vi "Auto_calibrate.vi"(3 "Mode":T4, 5 "Traverse line":T5 {"Row Duration (mins)" format="%#.1f"; "Row No" min=0; "Trace Gas Concentration (%)" min=0.0 format="%#.2f"; "Emission Rate (l/min)" format="%#.2f"; "Tunnel Speed" format="%#.2f"; "Start X" format="%#.2f"; "Start Y" format="%#.2f"; "Start Z" format="%#.2f"; "End X" format="%#.2f"; "End Y" format="%#.2f"; "End Z" format="%#.2f"; "Averaging time (min)" min=0.0 format="%#.2f"}) -> (0 "Error Messages":string, 1 "Status":T2, 2 "Traverse Out":T5 {"Row Duration (mins)" format="%#.1f"; "Row No" min=0; "Trace Gas Concentration (%)" min=0.0 format="%#.2f"; "Emission Rate (l/min)" format="%#.2f"; "Tunnel Speed" format="%#.2f"; "Start X" format="%#.2f"; "Start Y" format="%#.2f"; "Start Z" format="%#.2f"; "End X" format="%#.2f"; "End Y" format="%#.2f"; "End Z" format="%#.2f"; "Averaging time (min)" min=0.0 format="%#.2f"})   [LabVIEW 2014]
uses:
  Gen Trav/Traverse_cluster.ctl
  Gen Trav/Spacing.ctl
  Controls/Multi_run_mode.ctl
  Controls/User_Specific_mode.ctl
  Controls/Auto_Calib_Type.ctl
  Gen Trav/Multi_Run_Status.ctl
  Controls/Auto_Calib_Case.ctl
  File/Setup_Filetype.ctl
  Calibration/Calib_mode.ctl
  Controls/Setup.ctl
  Controls/Post_Process.ctl
  Controls/Save_Data.ctl
  ADAM Client/Sub VIs/ADAM Controls/Valco_valve_ph.ctl
  Controls/App_Global.ctl
  <vilib>/Analysis/baseanly.llb/Mean (DBL).vi
  Globals/Meas_global.vi
  Globals/Calib_global.vi
  Globals/Trav_pos_global.vi
  Globals/Extra_Commands_Global.vi
  <vilib>/Analysis/NI_AALBase.lvlib
panel:
  out "Minimum St Dev":dbl[](array[numeric])
  out "Time FFID valve moved":dbl
  out "Wait factor":dbl
  out "Establishment time":string
  out "Orig Calib file string":string
  out "Concentrations":dbl[](array[numeric])
  out "FFID St Dev":dbl[][](array[numeric]) format="%.2f"
  in  "Clear Calib History":bool
  out "Coefficients":dbl[][](array[numeric]) format="%.2f"
  out "Currently in Case":T1
  out "Valve position":dbl format="%.2f"
  out "Currently On":i32
  out "Values":dbl[][](array[numeric]) format="%.2f"
  out "FF Indexes":i16[](array[numeric])
  out "Ch No's":i16[](array[numeric])
  out "No of Calib Points":i32
  out "Root Name":string[](array[string])
  out "Calibration varying":T3
  in  "stop":bool
  out "New Calib Filenames":path[](array[path])
  # "Specific Argument Options\n      Tunnel Speed;1;2;3;4\nOR  Traverse Position\nOR   Concentration"
  # "X           Y            Z"
  # "Start"
  # "End"
  # "X           Y            Z"
  # "Start"
  # "End"
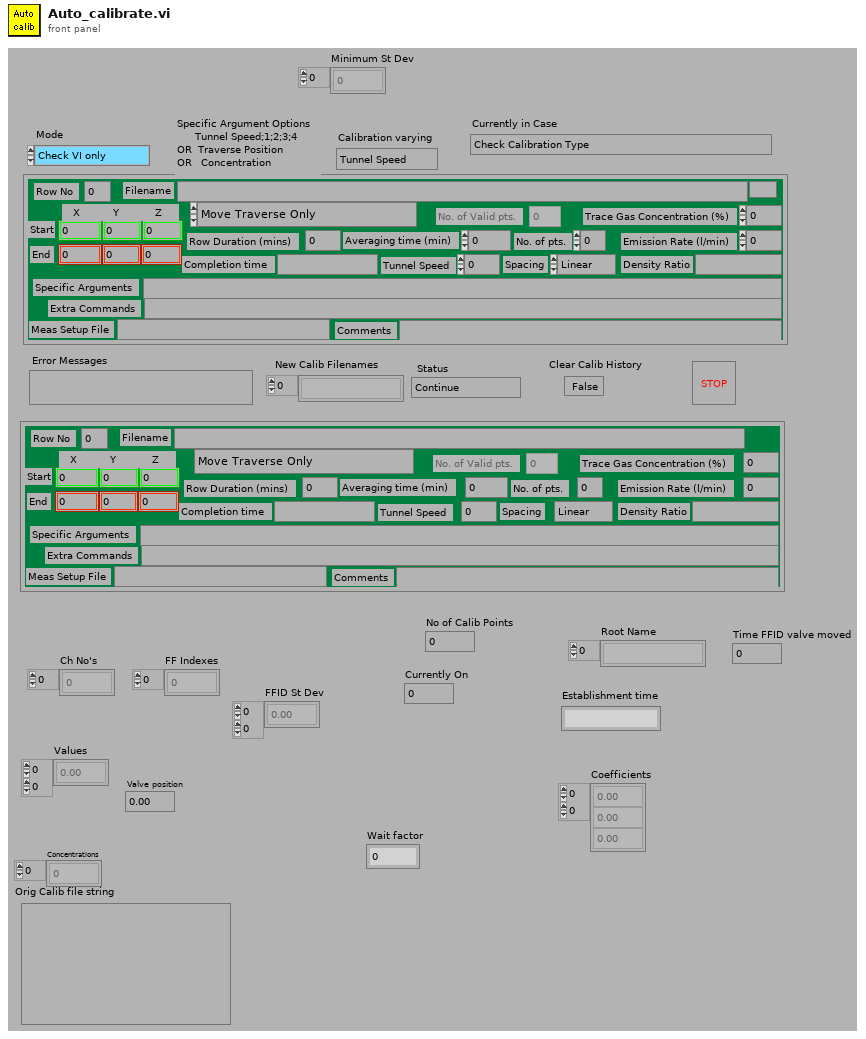
[diagram p1: front panel]
types:
  T1 = typedef "Auto_Calib_Case.ctl" = enum16{"Check Calibration Type", "Check if Original Calib file is Valid", "Get sampling rate etc. from meas setup file", "Setup Calibration Program", "Get Channel Numbers", "Check use latest selected on Mesurement setup files", "Create New Calib Filenames", "Setup Calibration Values in 2D array", "Create Measurement Setup File (Concentration Only)", "Are There Enough Calibration Points", "Set Measurement Conditions", "Measure Calibration Point", "Do Another Calibration Point?", "Skip Next Frame?", "Insert New calibration Filenames into Measurement Setup file", "Warn if FFID calibration is very non linear", "Warn if FFID variance is high", "Insert Bkgnd Variance into calib file", "Warn if FFID voltages are too low", "Warn if Current Calibration fit is poor", "Warn if Calibration Coefficients have significantly altered", "End"}
  T2 = typedef "Multi_Run_Status.ctl" = enum16{"Continue", "Jump to Next Point", "Jump to Next Row", "Jump To Fall Back", "Terminate Run"}
  T3 = typedef "Auto_Calib_Type.ctl" = enum16{"Tunnel Speed", "Traverse Position", "Concentration"}
  T4 = typedef "User_Specific_mode.ctl" = enum16{"Check VI only", "Run VI"}
  T5 = typedef "Traverse_cluster.ctl" = cluster{"Start X":dbl, "Start Y":dbl, "Start Z":dbl, "End X":dbl, "End Y":dbl, "End Z":dbl, "No. of pts.":i32, "Spacing":T6, "Filename":path, "Tunnel Speed":dbl, "Averaging time (min)":dbl, "Extra Commands":string, "Specific Arguments":string, "Emission Rate (l/min)":dbl, "Trace Gas Concentration (%)":dbl, "Density Ratio":string, "Comments":string, "Row No":i32, "Row Type Selector":T7, "Completion time":string, "Row Duration (mins)":dbl, "No. of Valid pts.":i32, "Meas Setup File":string}
  T6 = typedef "Spacing.ctl" = enum16{"Linear", "Log", "Gauss", "Specified", "N/A"}
  T7 = typedef "Multi_run_mode.ctl" = enum16{"Move Traverse Only", "Set Tunnel Speed Only", "Set Source Only", "Set Measurement Conditions", "Single Measurement", "Vertical Profile", "Lateral Profile", "Longitudinal Profile", "Explore Volume", "Multi-Axis Profile", "Auto Calibrate", "Meas Fast FID Bkgnd", "Check Beam Power", "Scanning Valve Measurement", "Run VI Named:", "Set ADAM Ch", "Wait (minutes)", "Send Message", "Synchronize With:", "Fall Back to this Row", "Turn Off Row Repeating", "Blank Row", "Traverse 3D Volume"}
  T8 = typedef "Setup_Filetype.ctl" = enum16{"Measurement Setups", "Calibration Setups", "General", "Results File Plotter Setups", "Speed Calib Tweaks"}
  T9 = typedef "Calib_mode.ctl" = enum16{"Show Setup", "Take a New Calibration Point", "Refit Curve", "Setup Front Panel"}
  T10 = typedef "Save_Data.ctl" = enum16{"Save No Data", "Save Data"}
  T11 = typedef "Post_Process.ctl" = enum16{"Take New Data", "Post Process Raw Data File"}
  T12 = typedef "Setup.ctl" = enum16{"Run Program", "Show Setup", "Save Current Setup", "Setup Front Panel"}
  T13 = typedef "App_Global.ctl" = enum16{"Read Global", "Write to Global", "Initialise Array"}
  T14 = typedef "Cal_Inst_type.ctl" = enum16{"Propeller anemometer", "Pressure Transducer", "Hot wire", "Cross wire velocity", "Cross wire angle", "Generic Linear", "Generic Polynomial", "Generic BackPoly", "Fast FID", "Thermocouple", "Cold wire", "Pulsed Wire"}
  T15 = typedef "Ref_Inst_type.ctl" = enum16{"Propellor anemometer", "Pressure Transducer", "Raw voltage", "Pitot-static tube", "Preston tube", "Generic Linear", "Generic Polynomial", "Thermocouple", "LDA", "Enter Value", "ADAM Channel"}
  T16 = cluster{"2nd Ref type":T15, "2nd inst present":bool}
  T17 = cluster{"high limit (10V)":sgl, "low limit (-10V)":sgl, "Ch No":i16, "Var name":string}[]
  T18 = cluster{"high limit (10V)":sgl, "low limit (-10V)":sgl, "Ch No":i16, "Var name":string}
  T19 = typedef "Inst_type.ctl" = enum16{"Propeller anemometer", "Raw voltage", "Pressure Transducer", "Pitot-static tube", "Preston tube", "Hot wire", "Cross wire 1", "Cross wire 2", "Generic Linear", "Generic Polynomial", "Generic BackPoly", "Fast FID", "Thermocouple", "Cold wire", "Pulsed Wire", "LDA Vel", "LDA Tran time", "LDA Arr time"}
  T20 = cluster{"high limit (10V)":sgl, "low limit (-10V)":sgl, "Ch No":i16, "Calib filename":path, "Inst type":T19, "Symbol":string, "Move channel":bool, "Use Latest":bool, "D":dbl, "Ch Name":string}[]
  T21 = typedef "Status_Cluster.ctl" = cluster{"Status":T2, "Error Type":string, "Error Description":string}
  T22 = typedef "Valco_valve_ph.ctl" = u16
  T23 = typedef "Time_Trace_Cluster.ctl" = cluster{"Weighting":dbl[], "Time (s)":dbl[], "Voltage":dbl[], "Eng Values":dbl[]}
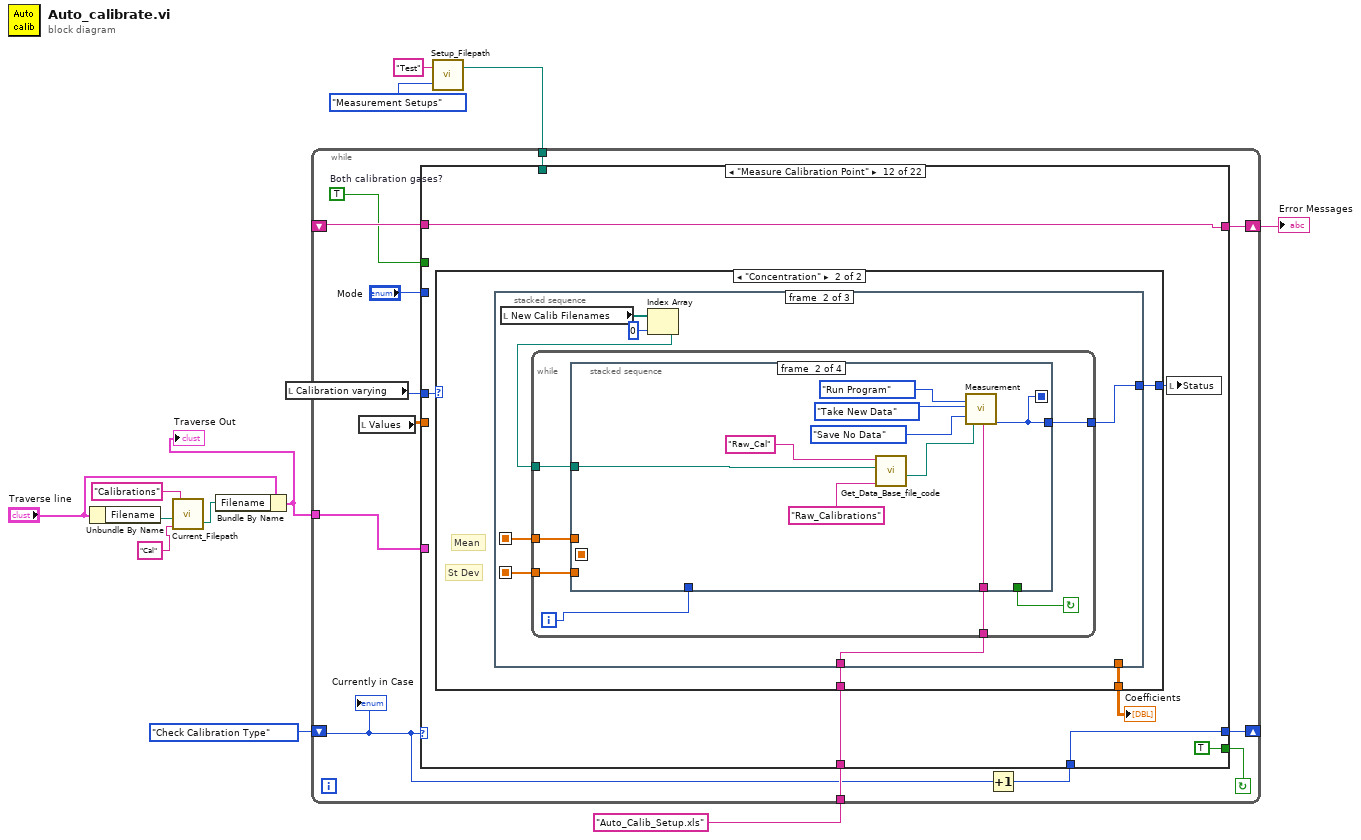
[diagram p0: block diagram]
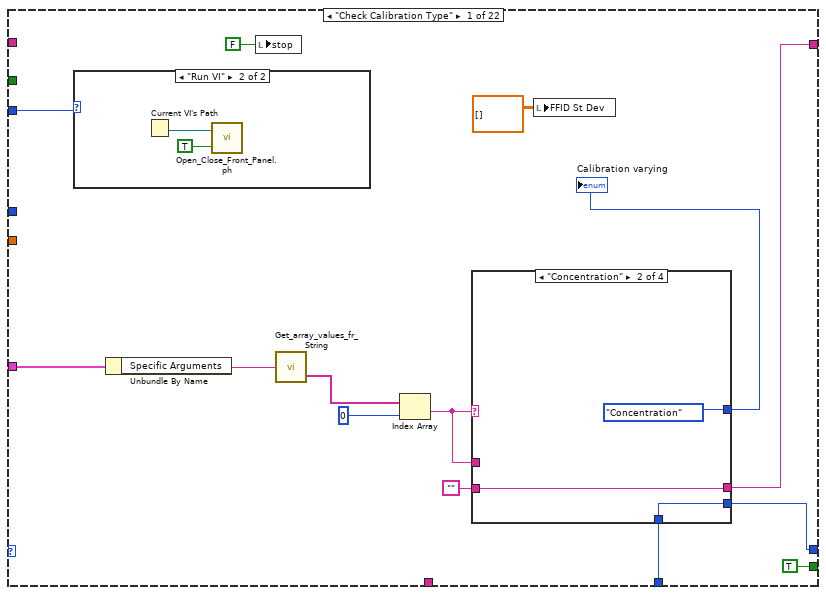
[diagram p2: hidden frame]
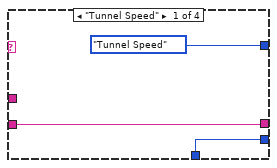
[diagram p4: hidden frame]
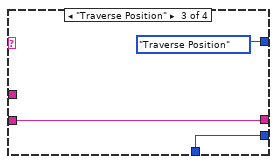
[diagram p5: hidden frame]
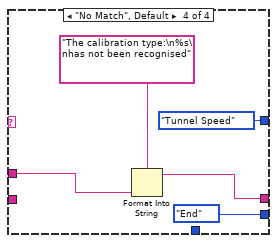
[diagram p6: hidden frame]
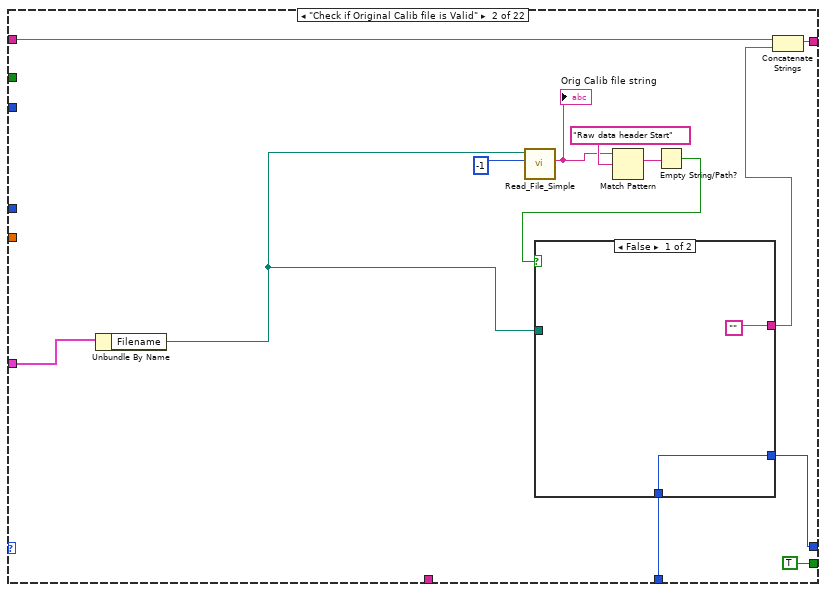
[diagram p7: hidden frame]
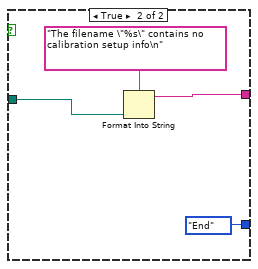
[diagram p8: hidden frame]
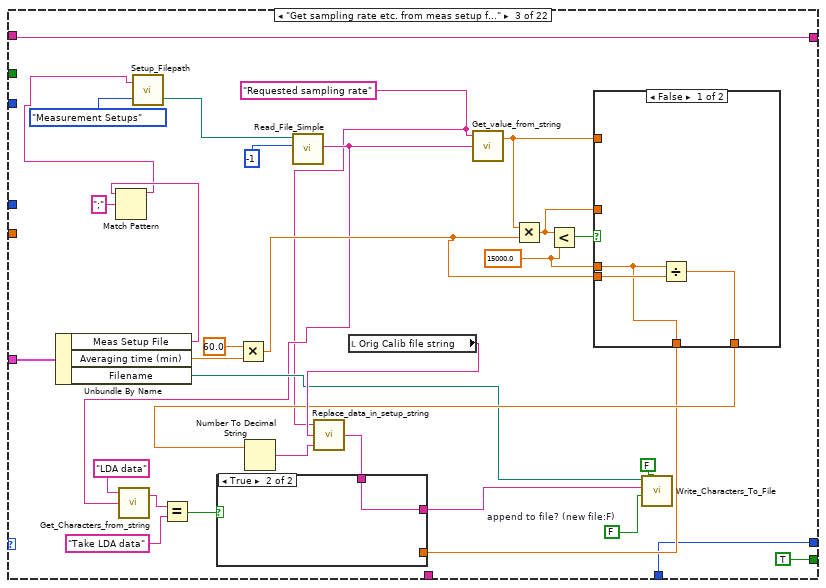
[diagram p9: hidden frame]
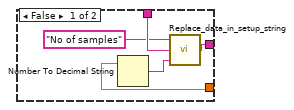
[diagram p10: hidden frame]
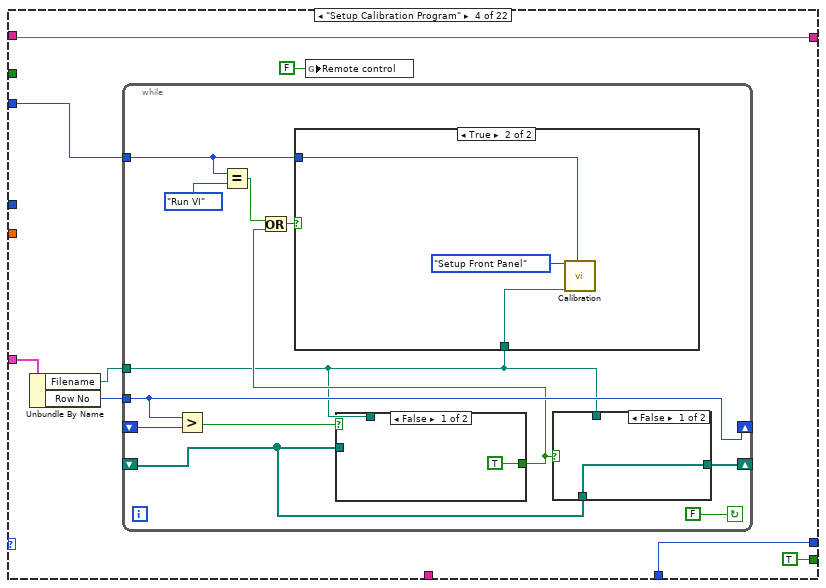
[diagram p12: hidden frame]
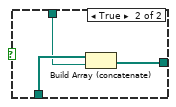
[diagram p13: hidden frame]
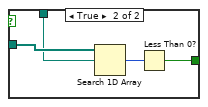
[diagram p15: hidden frame]
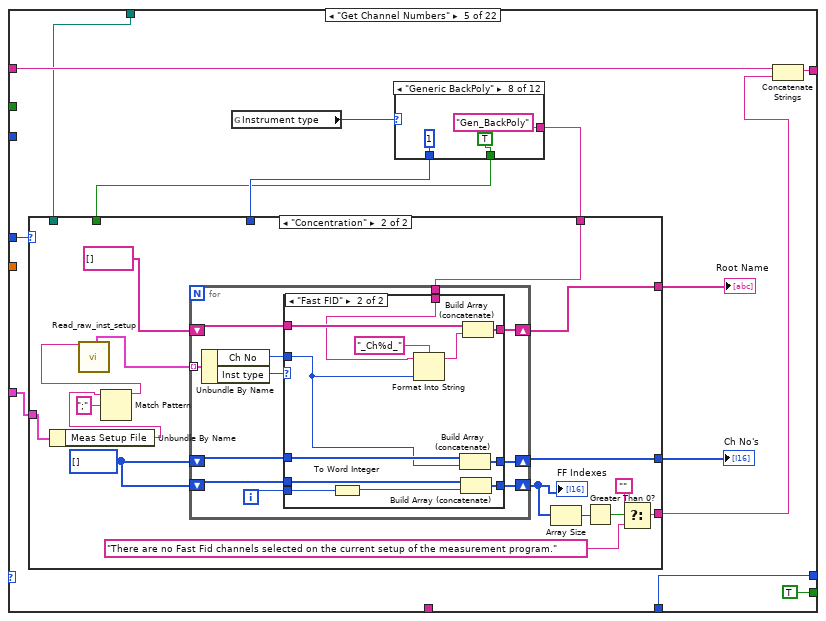
[diagram p16: hidden frame]
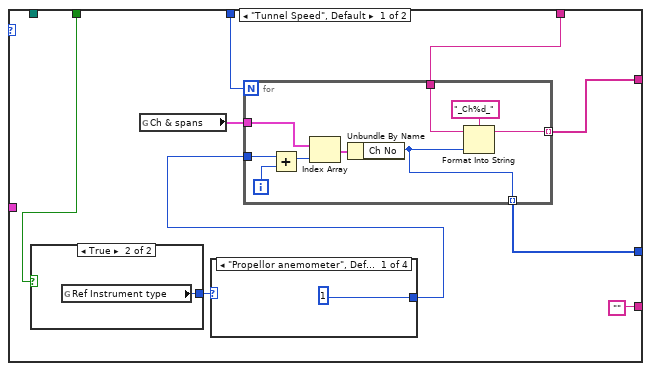
[diagram p17: hidden frame]
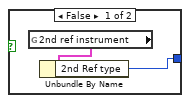
[diagram p18: hidden frame]
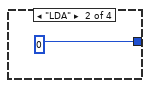
[diagram p19: hidden frame]
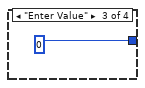
[diagram p20: hidden frame]
diagram:
  n1 = Unbundle By Name("Traverse line") -> ("Filename"=w5:path)
  n2 = call "Current_Filepath.vi"("Short_Name"="Cal" ("Data Type"), "Filename in"=w5, "Data Type"="Calibrations") -> ("Filename Out"=w4:path)  [unwired: 1 in, 1 out]
  n3 = Bundle By Name(cluster="Traverse line", "Filename"=w4) -> (w2:T5)
  "Traverse Out" <- w2
  n4 = call "Setup_Filepath.vi"("Setup File Type"=Setup_Filetype."Measurement Setups", "Filename in"="Test") -> ("Directory"=w7:path)  [unwired: 1 out]
  n5 = while {
    shift-left: _ -> [w18]
    shift-right: [w19] -> w11
    shift-left: Auto_Calib_Case."Check Calibration Type" ("Currently in Case") -> [w17]
    shift-right: [w16] -> _
    tunnel: "Auto_Calib_Setup.xls" -> [w25]
    tunnel: w7 -> [w14]
    tunnel: w2 -> [w13]
    stop <- w22 continue-if-true
    w15 = TRUE  # Both calibration gases?
    n6 = local read "Calibration varying"() -> (w21:T3)
    n7 = local read "Values"() -> (w20:dbl[][])
    n8 = Increment(x=w17) -> (x+1=w23:T1)
    n9 = case shown="\"Measure Calibration Point\"" w17 {
      tunnel: w13 -> [w39 w68 w106 w121 w152 _ w320 w375 w408 _ w575 _ _ _ _ _ _ _ _ _ w984 w1015]
      tunnel: "Mode" -> [w30 _ _ w122 _ _ w327 _ w409 _ w570 _ w728 _ _ _ _ _ _ _ _ w1016]
      tunnel: w25 -> [_ _ _ _ _ _ _ _ w413 _ _ w638 _ _ _ _ _ _ _ _ _ _]
      tunnel: [w28 w58 w88 w124 w155 w271 w324 w366 w411 w538 w563 w637 w729 w755 w767 w786 w824 w889 w907 w963 w1007 w1020] -> w16
      tunnel: w23 -> [w29 w57 w88 w124 w155 w271 w324 w367 w411 w537 w558 w637 _ w754 w766 w786 w824 w889 w907 w963 w1007 w1020]
      tunnel: [TRUE TRUE TRUE TRUE TRUE TRUE TRUE TRUE w407 TRUE TRUE TRUE TRUE TRUE TRUE TRUE TRUE TRUE TRUE TRUE TRUE FALSE] -> w22
      tunnel: w21 -> [_ _ _ _ w159 _ w323 w373 _ _ w562 w639 w727 w753 w769 _ _ _ _ _ _ w1017]
      tunnel: w20 -> [_ _ _ _ _ _ _ _ w406 w547 w574 _ _ _ _ _ w831 _ w913 _ _ _]
      tunnel: [w32 w60 w86 w125 w156 w272 w337 w370 w412 w541 w559 w635 w726 w758 w773 w795 w838 w885 w914 w952 w1000 w1019] -> w19
      tunnel: w18 -> [_ w62 w86 w125 w158 w272 w337 w369 w412 w542 w559 w635 w726 w758 w773 w795 w838 w885 w914 w952 w1000 w1019]
      tunnel: w15 -> [_ _ _ _ _ _ _ w368 _ _ _ _ _ _ _ _ _ _ _ _ _ w1014]
      tunnel: w14 -> [_ _ _ _ w151 w274 _ _ w410 _ _ _ _ _ _ _ _ _ _ _ _ _]
      frame "Check Calibration Type" {
        n10 = case shown="\"Run VI\"" w30 {
          frame "Check VI only" {
          }
          frame "Run VI" {
            n11 = Current VI's Path() -> (path=w40:path)
            n12 = call "Open_Close_Front_Panel.ph.vi"("Front Panel Window:Open"=TRUE, "VI path"=w40) -> ()  [unwired: 2 out]
          }
        }
        n13 = Unbundle By Name(w39) -> ("Specific Arguments"=w38:string)
        n14 = local write "stop"(FALSE) -> ()
        n15 = call "Get_array_values_fr_String.vi"("String Value"=w38) -> ("String array"=w37:string[])  [unwired: 1 out]
        n16 = Index Array(array=w37, index=0 ("Index")) -> (element=w35:string)
        n17 = case shown="\"Concentration\"" w35 {
          tunnel: [Auto_Calib_Type."Tunnel Speed" ("Calibration varying") Auto_Calib_Type."Concentration" ("Calibration varying") Auto_Calib_Type."Traverse Position" ("Calibration varying") Auto_Calib_Type."Tunnel Speed" ("Calibration varying")] -> w33
          tunnel: w35 -> [_ _ _ w54]
          tunnel: [w43 w46 w49 w52] -> w32
          tunnel: "" -> [w43 w46 w49 _]
          tunnel: w29 -> [w42 w45 w48 _]
          tunnel: [w42 w45 w48 Auto_Calib_Case."End" ("Currently in Case")] -> w28
          frame "Tunnel Speed" {
          }
          frame "Concentration" {
            (unwired) ""
          }
          frame "Traverse Position" {
          }
          frame "No Match", Default {
            n18 = Format Into String(format string="The calibration type:\n%s\nhas not been recognised" ("Format String"), w54) -> (resulting string=w52:string)  [unwired: 2 in, 1 out]
          }
        }
        "Calibration varying" <- w33
        n19 = local write "FFID St Dev"(dbl[][] [] ("FFID Variance")) -> ()
      }
      frame "Check if Original Calib file is Valid" {
        n20 = Unbundle By Name(w68) -> ("Filename"=w56:path)
        n21 = call "Read_File_Simple.vi"("Filename"=w56, "number of characters (all:-1)"=-1) -> ("string"=w65:string)  [unwired: 1 in, 7 out]
        "Orig Calib file string" <- w65
        n22 = Match Pattern(string=w65, regular expression="Raw data header Start") -> (match substring=w64:string)  [unwired: 4 out]
        n23 = Empty String/Path?(string/path=w64) -> (empty?=w63:bool)
        n24 = case shown="False" w63 {
          tunnel: w56 -> [_ w74]
          tunnel: ["" w72] -> w61
          tunnel: [w69 Auto_Calib_Case."End" ("Currently in Case")] -> w58
          tunnel: w57 -> [w69 _]
          frame False {
          }
          frame True {
            n25 = Format Into String(format string="The filename \"%s\" contains no calibration setup info\n" ("Format String"), w74) -> (resulting string=w72:string)  [unwired: 2 in, 1 out]
          }
        }
        n26 = Concatenate Strings(w62, w61) -> (w60:string)
      }
      frame "Get sampling rate etc. from meas setup file" {
        w89 = FALSE  # append to file? (new file:F)
        w78 = "Requested sampling rate"
        w96 = 15000.0 ("y")
        n27 = Unbundle By Name(w106) -> ("Meas Setup File"=w84:string, "Averaging time (min)"=w104:dbl, "Filename"=w91:path)
        n28 = Match Pattern(string=w84, regular expression=";") -> (before substring=w76:string)  [unwired: 4 out]
        n29 = call "Setup_Filepath.vi"("Setup File Type"=Setup_Filetype."Measurement Setups", "Filename in"=w76) -> ("Filename Out"=w75:path)  [unwired: 1 out]
        n30 = Multiply(x=60.0, y=w104) -> (x*y=w95:dbl)
        n31 = call "Read_File_Simple.vi"("Filename"=w75, "number of characters (all:-1)"=-1) -> ("string"=w83:string)  [unwired: 1 in, 7 out]
        n32 = call "Get_Characters_from_string.vi"("Input string"=w83, "Variable name"="LDA data") -> ("Value"=w81:string)  [unwired: 1 in, 1 out]
        n33 = Equal?(x=w81, y="Take LDA data") -> (x = y?=w79:bool)
        n34 = local read "Orig Calib file string"() -> (w100:string)
        n35 = call "Get_value_from_string.vi"("Input string"=w83, "Variable name"=w78) -> ("Value"=w99:dbl)  [unwired: 1 in, 1 out]
        n36 = Multiply(x=w99, y=w95) -> (x*y=w94:dbl)
        n37 = Less?(x=w94, y=w96) -> (x < y?=w102:bool)
        n38 = case shown="False" w102 {
          tunnel: w99 -> [_ w117]
          tunnel: [w114 w117] -> w98
          tunnel: w96 -> [w113 _]
          tunnel: w95 -> [w115 _]
          tunnel: [w113 w116] -> w92
          tunnel: w94 -> [_ w116]
          frame False {
            n39 = Divide(x=w113, y=w115) -> (x/y=w114:dbl)
          }
          frame True {
          }
        }
        n40 = Number To Decimal String(number=w98) -> (decimal integer string=w97:string)  [unwired: 1 out]
        n41 = call "Replace_data_in_setup_string.vi"("New data string"=w97, "Input string"=w100, "Variable name"=w78) -> ("Appended string"=w93:string)
        n42 = case shown="True" w79 {
          tunnel: w93 -> [w111 w112]
          tunnel: w92 -> [w108 _]
          tunnel: [w107 w112] -> w90
          frame False {
            n43 = Number To Decimal String(number=w108) -> (decimal integer string=w109:string)  [unwired: 1 out]
            n44 = call "Replace_data_in_setup_string.vi"("New data string"=w109, "Input string"=w111, "Variable name"="No of samples") -> ("Appended string"=w107:string)
          }
          frame True {
          }
        }
        n45 = call "Write_Characters_To_File.vi"("file path (dialog if empty)"=w91, "advisory dialog? (display:T)"=FALSE, "character string"=w90, "append to file? (new file:F)"=w89) -> ()  [unwired: 1 in, 4 out]
      }
      frame "Setup Calibration Program" {
        n46 = Unbundle By Name(w121) -> ("Filename"=w118:path, "Row No"=w120:i32)
        n47 = while {
          shift-left: _ -> [w129]
          shift-right: [w128] -> _
          tunnel: w120 -> [w136]
          shift-left: _ -> [w137]
          shift-right: [w136] -> _
          tunnel: w122 -> [w134]
          tunnel: w118 -> [w126]
          stop <- FALSE continue-if-true
          n48 = Greater?(x=w136, y=w137) -> (0:w135:bool)
          n49 = Equal?(x=w134, y=User_Specific_mode."Run VI" ("Mode")) -> (x = y?=w132:bool)
          n50 = case shown="False" w135 {
            tunnel: w129 -> [_ w149]
            tunnel: w126 -> [_ w148]
            tunnel: [TRUE w146] -> w130
            frame False {
            }
            frame True {
              n51 = Search 1D Array(1D array=w149, element=w148) -> (index of element=w147:i32)  [unwired: 1 out]
              n52 = Less Than 0?(x=w147) -> (x < 0?=w146:bool)
            }
          }
          n53 = Or(x=w132, y=w130) -> (x .or. y?=w131:bool)
          n54 = case shown="True" w131 {
            tunnel: w134 -> [_ w144]
            tunnel: w126 -> [_ w143]
            frame False {
            }
            frame True {
              n55 = call "Calibration.vi"("Mode"=Calib_mode."Setup Front Panel", "Calib file"=w143, "Simulate/Run"=w144) -> ()  [unwired: 17 out]
            }
          }
          n56 = case shown="False" w130 {
            tunnel: w129 -> [w138 w141]
            tunnel: w126 -> [_ w140]
            tunnel: [w138 w139] -> w128
            frame False {
            }
            frame True {
              n57 = Build Array (concatenate)(w141, w140) -> (w139:path[])
            }
          }
        }
        n58 = global write "Meas_global.vi" "Remote control"(FALSE ("Remote control")) -> ()
      }
      frame "Get Channel Numbers" {
        n59 = global read "Calib_global.vi" "Instrument type"() -> (w163:T14)
        n60 = case shown="\"Generic BackPoly\"" w163 {
          tunnel: ["Prop" "Mano" "HW" "XW" "XW" "Gen_Lin" "Gen_Poly" "Gen_BackPoly" "FF" "Therm" "CW" "PWA"] -> w162
          tunnel: [1 1 1 2 2 1 1 1 1 1 1 1] -> w153
          tunnel: [TRUE TRUE TRUE TRUE FALSE TRUE TRUE TRUE TRUE TRUE TRUE TRUE] -> w150
          frame "Propeller anemometer" {
          }
          frame "Pressure Transducer" {
          }
          frame "Hot wire" {
          }
          frame "Cross wire velocity" {
          }
          frame "Cross wire angle" {
          }
          frame "Generic Linear" {
          }
          frame "Generic Polynomial" {
          }
          frame "Generic BackPoly" {
          }
          frame "Fast FID" {
          }
          frame "Thermocouple" {
          }
          frame "Cold wire" {
          }
          frame "Pulsed Wire" {
          }
        }
        n61 = case shown="\"Concentration\"" w159 {
          tunnel: w162 -> [w170 w204]
          tunnel: [w166 w203] -> w161
          tunnel: [w167 w201] -> w160
          tunnel: ["" w194] -> w157
          tunnel: w153 -> [w168 _]
          tunnel: w152 -> [_ w193]
          tunnel: w151 -> [_ _]
          tunnel: w150 -> [w164 _]
          frame "Tunnel Speed", Default {
            n62 = case shown="True" w164 {
              tunnel: [w173 w175] -> w172
              frame False {
                n63 = global read "Calib_global.vi" "2nd ref instrument"() -> (w174:T16)
                n64 = Unbundle By Name(w174) -> ("2nd Ref type"=w173:T15)
              }
              frame True {
                n65 = global read "Calib_global.vi" "Ref Instrument type"() -> (w175:T15)
              }
            }
            n66 = global read "Calib_global.vi" "Ch & spans"() -> (w169:T17)
            n67 = case shown="\"Propellor anemometer\", Default" w172 {
              tunnel: [1 i16 0 0 0] -> w165
              frame "Propellor anemometer", Default {
              }
              frame "LDA" {
              }
              frame "Enter Value" {
              }
              frame "ADAM Channel" {
              }
            }
            n68 = for {
              N: w168 -> [_]
              tunnel: [w182] -> w167 mode=indexing
              tunnel: w170 -> [w181]
              tunnel: w169 -> [w180]
              tunnel: [w179] -> w166 mode=indexing
              tunnel: w165 -> [w177]
              i -> [w178]
              n69 = Add(x=w177, y=w178) -> (x+y=w176:i32)
              n70 = Index Array(array=w180, index=w176) -> (element=w184:T18)
              n71 = Unbundle By Name(w184) -> ("Ch No"=w182:i16)
              n72 = Format Into String(format string="_Ch%d_" ("Format String"), initial string=w181, w182) -> (resulting string=w179:string)  [unwired: 1 in, 1 out]
            }
          }
          frame "Concentration" {
            w200 = i16[] []
            n73 = Unbundle By Name(w193) -> ("Meas Setup File"=w190:string)
            n74 = Match Pattern(string=w190, regular expression=";") -> (before substring=w189:string)  [unwired: 4 out]
            n75 = call "Read_raw_inst_setup.vi"("Setup file"=w189) -> ("Ch & spans choices"=w192:T20)  [unwired: 18 out]
            n76 = for {
              tunnel: w192 -> [w215] mode=indexing
              tunnel: w204 -> [w214]
              shift-right: [w210] -> w203
              shift-left: string[] [] -> [w211]
              shift-right: [w208] -> w201
              shift-left: w200 -> [w209]
              shift-right: [w207] -> w199
              shift-left: w200 -> [w206]
              i -> [w205]
              n77 = Unbundle By Name(w215) -> ("Ch No"=w213:i16, "Inst type"=w212:T19)
              n78 = case shown="\"Fast FID\"" w212 {
                tunnel: w214 -> [_ w220]
                tunnel: w213 -> [_ w222]
                tunnel: w211 -> [w218 w230]
                tunnel: [w218 w229] -> w210
                tunnel: w209 -> [w217 w228]
                tunnel: [w217 w227] -> w208
                tunnel: w206 -> [w216 w225]
                tunnel: [w216 w226] -> w207
                tunnel: w205 -> [_ w224]
                frame "Generic Linear", Default {
                }
                frame "Fast FID" {
                  n79 = To Word Integer(number=w224) -> (16bit integer=w223:i16)
                  n80 = Format Into String(format string="_Ch%d_", initial string=w220, w222) -> (resulting string=w219:string)  [unwired: 1 in, 1 out]
                  n81 = Build Array (concatenate)(w228, w222) -> (w227:i16[])
                  n82 = Build Array (concatenate)(w225, w223) -> (w226:i16[])
                  n83 = Build Array (concatenate)(w230, w219) -> (w229:string[])
                }
              }
            }
            "FF Indexes" <- w199
            n84 = Array Size(array=w199) -> (size(s)=w198:i32)
            n85 = Greater Than 0?(x=w198) -> (x > 0?=w197:bool)
            n86 = Select(t="", s=w197, f="There are no Fast Fid channels selected on the current setup of the measurement program.") -> (s? t:f=w194:string)
          }
        }
        "Root Name" <- w161
        "Ch No's" <- w160
        n87 = Concatenate Strings(w158, w157) -> (w156:string)
      }
      frame "Check use latest selected on Mesurement setup files" {
        n88 = global read "Trav_pos_global.vi" "Measurement setup files"() -> (w267:string[])
        n89 = local read "Ch No's"() -> (w273:i16[])
        n90 = Build Array (concatenate)(w267, "Current_Setup.xls") -> (w268:string[])
        n91 = for {
          tunnel: w274 -> [w277]
          tunnel: w268 -> [w276] mode=indexing
          tunnel: w273 -> [w275]
          n92 = stacked-sequence {
            seq-local: [w278 _ _] -> [_ w284 w312]
            seq-local: [_ w282 _] -> [_ _ w310]
            tunnel: w277 -> [w281 _ w309]
            tunnel: w276 -> [w280 _ w308]
            tunnel: w275 -> [_ w283 _]
            frame #0 {
              n93 = Build Path(base path=w281, name or relative path=w280) -> (appended path=w279:path)
              n94 = call "Read_File_Simple.vi"("Filename"=w279) -> ("string"=w278:string)  [unwired: 2 in, 7 out]
            }
            frame #1 {
              n95 = while {
                shift-right: [w289] -> w282
                shift-left: w284 -> [w290]
                tunnel: w283 -> [w293]
                i -> [w297]
                stop <- w286 continue-if-true
                n96 = Increment(x=w297) -> (x+1=w291:i32)
                n97 = Format Into String(format string="An ch %d Ch No", w291) -> (resulting string=w296:string)  [unwired: 2 in, 1 out]
                n98 = call "Get_value_from_string.vi"("Input string"=w290, "Variable name"=w296) -> ("Status"=w295:enum16{"Char in string", "Char not in string"}, "Value"=w294:dbl)  [unwired: 1 in]
                n99 = To Long Integer(number=w294) -> (32bit integer=w292:i32)
                n100 = Search 1D Array(1D array=w293, element=w292) -> (index of element=w288:i32)  [unwired: 1 in]
                n101 = Greater Or Equal To 0?(x=w288) -> (x >= 0?=w287:bool)
                n102 = case shown="\"Char in string\"" w295 {
                  tunnel: [TRUE FALSE] -> w286
                  frame "Char in string" {
                  }
                  frame "Char not in string" {
                  }
                }
                n103 = And(x=w287, y=w286) -> (x .and. y?=w285:bool)
                n104 = case shown="True" w285 {
                  tunnel: w291 -> [w301 _]
                  tunnel: w290 -> [w300 w305]
                  tunnel: [w299 w305] -> w289
                  frame True {
                    n105 = Format Into String(format string="An ch %d Use latest Calib", w301) -> (resulting string=w303:string)  [unwired: 2 in, 1 out]
                    n106 = call "Replace_data_in_setup_string.vi"("New data string"="TRUE" ("Replace with"), "Input string"=w300, "Variable name"=w303) -> ("Appended string"=w299:string)
                  }
                  frame False {
                  }
                }
              }
            }
            frame #2 {
              n107 = Equal?(x=w312, y=w310) -> (x = y?=w311:bool)
              n108 = case shown="True" w311 {
                tunnel: w309 -> [w315 _]
                tunnel: w310 -> [w318 _]
                tunnel: w308 -> [w314 _]
                frame False {
                  w317 = FALSE  # append to file? (new file:F)
                  n109 = Build Path(base path=w315, name or relative path=w314) -> (appended path=w313:path)
                  n110 = call "Write_Characters_To_File.vi"("file path (dialog if empty)"=w313, "advisory dialog? (display:T)"=FALSE, "character string"=w318, "append to file? (new file:F)"=w317) -> ()  [unwired: 1 in, 4 out]
                }
                frame True {
                }
              }
            }
          }
        }
      }
      frame "Create New Calib Filenames" {
        n111 = Unbundle By Name(w320) -> ("Filename"=w319:path)
        n112 = Get Date/Time String(date format (0)=enum16{"short", "long", "abbreviated"}."short") -> (date string=w331:string)  [unwired: 3 out]
        n113 = Strip Path(path=w319) -> (stripped path=w326:path)  [unwired: 1 out]
        n114 = local read "Root Name"() -> (w322:string[])
        n115 = case shown="\"Tunnel Speed\", Default" w323 {
          tunnel: w322 -> [_ w342]
          tunnel: [1 w341] -> w321
          frame "Tunnel Speed", Default {
          }
          frame "Concentration" {
            n116 = Array Size(array=w342) -> (size(s)=w341:i32)
          }
        }
        n117 = call "Replace_Character.vi"("Replace with"="-", "Input String"=w331, "Search For"="/") -> ("Output string"=w328:string)  [unwired: 1 out]
        n118 = List Folder(path=w326) -> (filenames=w339:string[])  [unwired: 1 in, 5 out]
        n119 = To Upper Case(1:w339) -> (0:w338:string[])
        n120 = for {
          N: w321 -> [_]
          tunnel: w322 -> [w345] mode=indexing
          tunnel: w338 -> [w349]
          tunnel: w326 -> [w348]
          tunnel: [w344] -> w335 mode=indexing
          tunnel: w328 -> [w346]
          tunnel: w327 -> [w343]
          n121 = while {
            tunnel: w345 -> [w356]
            tunnel: w346 -> [w357]
            tunnel: [w352] -> w347
            tunnel: w349 -> [w359]
            i -> [w361]
            stop <- w363 continue-if-true
            n122 = Increment(x=w361) -> (x+1=w358:i32)
            n123 = Format Into String(format string="%s_%d.xls" ("Format String"), initial string=w356, w357, w358) -> (resulting string=w353:string)  [unwired: 1 in, 1 out]
            n124 = call "Replace_Character.vi"("Replace with"="_", "Input String"=w353, "Search For"=" ") -> ("Output string"=w352:string)  [unwired: 1 out]
            n125 = To Upper Case(1:w352) -> (0:w362:string)
            n126 = Search 1D Array(1D array=w359, element=w362) -> (index of element=w364:i32)  [unwired: 1 out]
            n127 = Not Equal?(x=w364, y=-1) -> (x != y?=w363:bool)
          }
          n128 = Build Path(base path=w348, name or relative path=w347) -> (appended path=w344:path)
          n129 = case shown="\"Run VI\"" w343 {
            tunnel: w344 -> [_ w350]
            frame "Check VI only" {
            }
            frame "Run VI" {
              n130 = call "Calibration.vi"("Mode"=Calib_mode."Setup Front Panel", "Calib file"=w350) -> ()  [unwired: 1 in, 17 out]
            }
          }
        }
        "New Calib Filenames" <- w335
        n131 = Index Array(array=w335, index=0 ("Index")) -> (element=w333:path)
        n132 = global write "Meas_global.vi" "Results file"(w333) -> ()
        "Establishment time" <- "!Establish Exp Conditions (s) = 15" ("Message")
      }
      frame "Setup Calibration Values in 2D array" {
        n133 = case shown="\"Concentration\"" w373 {
          tunnel: [w384 w390 w405] -> w372
          tunnel: w375 -> [w379 _ w404]
          tunnel: ["" "" w403] -> w371
          tunnel: w368 -> [_ w388 _]
          tunnel: w367 -> [w378 w387 w402]
          tunnel: [w377 w387 w401] -> w366
          frame "Tunnel Speed" {
            n134 = Unbundle By Name(w379) -> ("Specific Arguments"=w382:string)
            n135 = call "Get_array_values_fr_String.vi"("String Value"=w382) -> ("Numeric Array"=w380:dbl[])  [unwired: 1 out]
            n136 = Array Subset(array=w380, index=1 ("Array Index")) -> (w376:dbl[])  [unwired: 1 in]
            n137 = for {
              tunnel: w376 -> [w386] mode=indexing
              tunnel: [w385] -> w384 mode=indexing
              n138 = Build Array(w386) -> (w385:dbl[])
            }
            n139 = Increment(x=w378) -> (x+1=w377:T1)
          }
          frame "Concentration" {
            n140 = case shown="True" w388 {
              tunnel: [w392 w396] -> w391
              frame True {
                n141 = Build Array(1.0, 2.0, 3.0) -> (w392:dbl[])
              }
              frame False {
                n142 = Build Array(1.0, 3.0) -> (w396:dbl[])
              }
            }
            n143 = for {
              tunnel: w391 -> [w400] mode=indexing
              tunnel: [w399] -> w390 mode=indexing
              n144 = Build Array(w400) -> (w399:dbl[])
            }
          }
          frame "Traverse Position" {
            n145 = call "Create_Pos_array.vi"("Traverse line"=w404) -> ("Error Messages"=w403:string, "Array of Positions"=w405:dbl[][])  [unwired: 5 in, 2 out]
            n146 = Increment(x=w402) -> (x+1=w401:T1)
          }
        }
        "Values" <- w372
        n147 = Concatenate Strings(w369, w371) -> (w370:string)
      }
      frame "Create Measurement Setup File (Concentration Only)" {
        n148 = stacked-sequence {
          seq-local: [w424 _ _ _ _ _] -> [_ w443 _ _ _ _]
          seq-local: [_ w441 _ _ _ _] -> [_ _ w464 _ _ _]
          tunnel: w410 -> [w415 _ w465 _ _ _]
          tunnel: w413 -> [_ _ w466 _ _ _]
          tunnel: w409 -> [_ _ _ _ w479 w522]
          tunnel: w408 -> [w421 _ _ _ w489 _]
          tunnel: [_ _ _ _ w488 _] -> w407
          tunnel: w406 -> [_ _ _ _ w482 _]
          frame #0 {
            w428 = TRUE  # Show Dialog?
            n149 = Unbundle By Name(w421) -> ("Meas Setup File"=w422:string)
            n150 = Match Pattern(string=w422, regular expression=";") -> (before substring=w420:string)  [unwired: 4 out]
            n151 = Build Path(base path=w415, name or relative path=w420) -> (appended path=w429:path)
            n152 = Format Into String(format string="Meas Setup File   %s", w415) -> (resulting string=w414:string)  [unwired: 2 in, 1 out]
            n153 = call "Read_spec_No_of_Characters.vi"("Filename"=w429) -> ("character string"=w430:string)  [unwired: 1 out]
            n154 = call "Get_string_subset.vi"("String Name"=w414, "Show Dialog?"=w428, "String to split"=w430, "File Label"="Raw data header") -> ("Output string"=w417:string)  [unwired: 1 out]
            n155 = call "Get_value_from_string.vi"("Input string"=w417, "Variable name"="No of analogue inst") -> ("Value"=w418:dbl)  [unwired: 1 in, 1 out]
            n156 = for {
              N: w418 -> [_]
              shift-right: [w432] -> w427
              shift-left: w417 -> [w434]
              i -> [w438]
              n157 = Increment(x=w438) -> (x+1=w437:i32)
              n158 = Number To Decimal String(number=w437) -> (decimal integer string=w440:string)  [unwired: 1 out]
              n159 = Concatenate Strings("An ch ", w440, " Inst type") -> (w435:string)
              n160 = call "Replace_data_in_setup_string.vi"("New data string"="Raw voltage", "Input string"=w434, "Variable name"=w435) -> ("Appended string"=w432:string)
            }
            n161 = call "Replace_data_in_setup_string.vi"("New data string"="No LDA data", "Input string"=w427, "Variable name"="LDA data" ("Label for characters")) -> ("Appended string"=w424:string)
          }
          frame #1 {
            n162 = global read "Calib_global.vi" "New Setup String"() -> (w444:string)
            n163 = for {
              N: 4 -> [_]
              shift-right: [w449] -> w441
              shift-left: w443 -> [w450]
              tunnel: w444 -> [w446]
              i -> [w448]
              n164 = case shown="3" w448 {
                tunnel: [w453 w456 w459 "No of blocks"] -> w447
                tunnel: w446 -> [w452 w455 w458 _]
                tunnel: [w451 w454 w457 "1" ("Value")] -> w445
                frame 0, Default {
                  w453 = "No of samples"
                  n165 = call "Get_Characters_from_string.vi"("Input string"=w452, "Variable name"=w453) -> ("Value"=w451:string)  [unwired: 1 in, 1 out]
                }
                frame 2 {
                  w456 = "Actual sampling rate"
                  n166 = call "Get_Characters_from_string.vi"("Input string"=w455, "Variable name"=w456) -> ("Value"=w454:string)  [unwired: 1 in, 1 out]
                }
                frame 3 {
                  w459 = "Board type"
                  n167 = call "Get_Characters_from_string.vi"("Input string"=w458, "Variable name"=w459) -> ("Value"=w457:string)  [unwired: 1 in, 1 out]
                }
                frame 1 {
                }
              }
              n168 = call "Replace_data_in_setup_string.vi"("New data string"=w445, "Input string"=w450, "Variable name"=w447) -> ("Appended string"=w449:string)
            }
          }
          frame #2 {
            w470 = FALSE  # advisory dialog? (display:T)
            w471 = FALSE  # append to file? (new file:F)
            n169 = call "Remove_Plug_Ins_etc.vi"("Input String"=w464) -> ("Output string"=w463:string)
            n170 = call "Add_label_to_string.vi"("String to write"=w463, "File Label"="Raw data header") -> ("Output string"=w467:string)
            n171 = Build Path(base path=w465, name or relative path=w466) -> (appended path=w462:path)
            n172 = call "Add_length_to_string.vi"("String in"=w467) -> ("String out"=w469:string)
            n173 = call "Write_Characters_To_File.vi"("file path (dialog if empty)"=w462, "advisory dialog? (display:T)"=w470, "character string"=w469, "append to file? (new file:F)"=w471) -> ()  [unwired: 1 in, 4 out]
          }
          frame #3 {
            w475 = 0.0 ("Input Element")
            n174 = Build Array("GMU:Calibration:Gas 1", "GMU:Calibration:Gas 2") -> (w477:string[])
            n175 = call "Get_Current_Scan_client.vi"("ADAM Ch Names"=w477) -> ("Numerical Values"=w476:dbl[])  [unwired: 3 out]
            n176 = Build Array (concatenate)(w475, w475, w476, w475) -> (→"Concentrations":dbl[])
          }
          frame #4 {
            w483 = 0 ("Index")
            w485 = dbl[] [20.0, 0.0, 0.0, 0.0]  # X Offset
            w487 = dbl[] [100.0, 30.0, 15.0, 0.0]  # Z Offset
            n177 = Index Array(array=w482, index (row)=w483, index (col)=w483) -> (element=w481:dbl)
            n178 = Unbundle By Name(w489) -> ("Start X"=w484:dbl, "Start Z"=w486:dbl)
            n179 = Equal?(x=User_Specific_mode."Run VI" ("Mode"), y=w479) -> (x = y?=w478:bool)
            n180 = for {
              tunnel: w479 -> [w507]
              tunnel: w489 -> [w511]
              tunnel: w487 -> [w510] mode=indexing
              tunnel: w486 -> [w508]
              tunnel: [w503] -> w488
              tunnel: w485 -> [w502] mode=indexing
              tunnel: w484 -> [w501]
              tunnel: w481 -> [w498]
              tunnel: w478 -> [w496]
              i -> [w493]
              stop <- w503 continue-if-true
              n181 = Greater?(x=w493, y=1) -> (0:w492:bool)
              n182 = Add(x=w501, y=w502) -> (x+y=w500:dbl)
              n183 = Add(x=w508, y=w510) -> (x+y=w509:dbl)
              n184 = Equal?(x=0, y=w493) -> (x = y?=w495:bool)
              n185 = And(x=w496, y=w495) -> (x .and. y?=w497:bool)
              n186 = case shown="True" w492 {
                tunnel: ["" "No Backlash"] -> w491
                tunnel: [1.0 ("f") 0.1 ("t")] -> w490
                frame False {
                }
                frame True {
                }
              }
              n187 = Bundle By Name(cluster=w511, "Start X"=w500, "Start Z"=w509, "Specific Arguments"=w491) -> (w512:T5)
              n188 = case shown="True" w497 {
                tunnel: w498 -> [_ w520]
                frame False {
                }
                frame True {
                  n189 = call "Fast_FID_Valve_Control.vi"("Requested Position"=w520) -> ()  [unwired: 7 out]
                  n190 = Get Date/Time In Seconds() -> (seconds since 1Jan1904=w519:timestamp)
                  n191 = To Double Precision Float(number=w519) -> (double precision float=→"Time FFID valve moved":dbl)
                }
              }
              n192 = call "Set_Traverse_Position.vi"("Simulate/Run"=w507, "Currently on Point"=1, "Traverse line"=w512) -> ("Status Cluster"=w504:T21)  [unwired: 2 out]
              n193 = Unbundle By Name(w504) -> ("Status"=w505:T2)
              n194 = global write "Trav_pos_global.vi" "Speed Factor"(w490) -> ()
              n195 = call "Prog_Status_Handler.vi"("Status Cluster"=w504, "Simulate/Run"=w507) -> ()  [unwired: 2 out]
              n196 = local write "Status"(w505) -> ()
              n197 = Equal?(x=w505, y=Multi_Run_Status."Continue" ("Status")) -> (x = y?=w503:bool)
            }
          }
          frame #5 {
            n198 = case shown="\"Run VI\"" w522 {
              frame "Check VI only", Default {
              }
              frame "Run VI" {
                n199 = while {
                  shift-right: [w534] -> _
                  shift-left: _ -> [w535]
                  tunnel: [w533] -> w528
                  stop <- TRUE stop-if-true
                  n200 = Get Date/Time In Seconds() -> (seconds since 1Jan1904=w534:timestamp)
                  n201 = Subtract(x=w534, y=w535) -> (x-y=w533:dbl)
                }
                n202 = Divide(x=w528, y=3600.0) -> (x/y=w527:dbl)
                n203 = Multiply(x=w527, y=0.2) -> (x*y=w525:dbl)
                n204 = Add(x=w525, y=0.8) -> (x+y=w523:dbl)
                n205 = In Range and Coerce(upper limit=2.0, x=w523, lower limit=1.0) -> (coerced(x)=→"Wait factor":dbl)  [unwired: 1 out]
              }
            }
            n206 = global write "Trav_pos_global.vi" "Speed Factor"(1.0 ("Speed Factor")) -> ()
          }
        }
      }
      frame "Are There Enough Calibration Points" {
        n207 = Array Size(array=w547) -> (size(s)=w548:i32[])
        n208 = Index Array(array=w548, index=0 ("Index")) -> (element=w543:i32)
        "No of Calib Points" <- w543
        n209 = Greater?(x=w543, y=1) -> (0:w544:bool)
        n210 = case shown="False" w544 {
          tunnel: ["Less than two calibration points have been specified\n" ""] -> w540
          tunnel: [Auto_Calib_Case."End" ("Currently in Case") w552] -> w538
          tunnel: w537 -> [_ w552]
          frame False {
          }
          frame True {
          }
        }
        n211 = Concatenate Strings(w542, w540) -> (w541:string)
        "Currently On" <- 1 ("Currently On")
      }
      frame "Set Measurement Conditions" {
        n212 = local read "Currently On"() -> (w554:i32)
        n213 = Decrement(x=w554) -> (x-1=w573:i32)
        n214 = Index Array(array=w574, index (row)=w573) -> (element=w572:dbl[])  [unwired: 1 in]
        n215 = case shown="\"Concentration\"" w562 {
          tunnel: w572 -> [w590 w607 w625]
          tunnel: w570 -> [_ _ w623]
          tunnel: w575 -> [w588 w603 w615]
          tunnel: [w589 w602 w613] -> w557
          tunnel: w554 -> [w584 _ w612]
          tunnel: [w587 w601 w619] -> w555
          frame "Tunnel Speed" {
            n216 = Index Array(array=w590, index=0 ("Index")) -> (element=w577:dbl)
            n217 = while {
              shift-right: [w598] -> w579
              shift-left: _ -> [w597]
              tunnel: w577 -> [w600]
              tunnel: [w598] -> w586
              tunnel: [w597] -> w585
              stop <- FALSE continue-if-true
              n218 = Greater Than 0?(x=w600) -> (x > 0?=w598:bool)
            }
            n219 = Exclusive Or(1:w585, 2:w586) -> (0:w582:bool)
            n220 = Greater?(x=w584, y=1) -> (0:w581:bool)
            n221 = And(x=w582, y=w581) -> (x .and. y?=w580:bool)
            n222 = case shown="False" w579 {
              tunnel: [w592 w594] -> w578
              tunnel: w577 -> [w593 w594]
              frame False {
                n223 = Negate(x=w593) -> (-x=w592:dbl)
              }
              frame True {
              }
            }
            n224 = case shown="True" w580 {
              frame False {
              }
              frame True {
                n225 = call "Wait_Seconds_with_display.vi"("Message"="Please rotate the probe you are calibrating", "Seconds to wait"=10000.0) -> ()  [unwired: 2 out]
              }
            }
            n226 = local read "Establishment time"() -> (w587:string)
            n227 = Bundle By Name(cluster=w588, "Tunnel Speed"=w578) -> (w589:T5)
          }
          frame "Traverse Position" {
            n228 = Index Array(array=w607, index=0 ("Index")) -> (element=w606:dbl)
            n229 = Index Array(array=w607, index=1 ("Index")) -> (element=w605:dbl)
            n230 = Index Array(array=w607, index=2 ("Index")) -> (element=w604:dbl)
            n231 = local read "Establishment time"() -> (w601:string)
            n232 = Bundle By Name(cluster=w603, "Start X"=w606, "Start Y"=w605, "Start Z"=w604) -> (w602:T5)
          }
          frame "Concentration" {
            w614 = nan ("Start X")
            n233 = Index Array(array=w625, index=0 ("Index")) -> (element=w616:dbl)
            n234 = case shown="2, Default" w612 {
              tunnel: [0.0 20.0] -> w611
              frame 1 {
              }
              frame 2, Default {
              }
            }
            n235 = local read "Wait factor"() -> (w618:dbl)
            n236 = case shown="\"Check VI only\"" w623 {
              tunnel: w616 -> [w630 w631]
              tunnel: [w629 w632] -> w624
              frame "Check VI only" {
                n237 = To Long Integer(number=w630) -> (32bit integer=w629:i32)
              }
              frame "Run VI" {
                n238 = call "Fast_FID_Valve_Control.vi"("Requested Position"=w631) -> ("Achieved Posn."=w632:T22)  [unwired: 6 out]
              }
            }
            n239 = Multiply(x=w618, y=w611) -> (x*y=w617:dbl)
            n240 = Number To Decimal String(number=w617) -> (decimal integer string=w620:string)  [unwired: 1 out]
            n241 = Concatenate Strings("!Establish Exp Conditions (s) = " ("Message"), w620) -> (w619:string)
            n242 = To Double Precision Float(number=w624) -> (double precision float=→"Valve position":dbl)
            n243 = Bundle By Name(cluster=w615, "Start X"=w614, "Start Y"=w614, "Start Z"=w614) -> (w613:T5)
          }
        }
        n244 = call "Add_Extra_Command.vi"("Traverse line"=w557, "Extra Command"=w555) -> ("Traverse line Out"=w556:T5)
        n245 = call "Set_Measurement_Conditions.vi"("Simulate/Run"=w570, "Currently on Point"=1, "Traverse line"=w556) -> ("Status Cluster"=w561:T21)  [unwired: 2 out]
        n246 = Unbundle By Name(w561) -> ("Status"=w560:T2)
        "Status" <- w560
        n247 = Equal?(x=w560, y=Multi_Run_Status."Continue" ("Status")) -> (x = y?=w566:bool)
        n248 = Equal?(x=User_Specific_mode."Run VI" ("Mode"), y=w570) -> (x = y?=w567:bool)
        n249 = Increment(x=w558) -> (x+1=w564:T1)
        n250 = And(x=w566, y=w567) -> (x .and. y?=w565:bool)
        n251 = Select(t=w558, s=w565, f=w564) -> (s? t:f=w563:T1)
      }
      frame "Measure Calibration Point" {
        n252 = case shown="\"Concentration\"" w639 {
          tunnel: w638 -> [_ w648]
          tunnel: [w642 w647] -> w634
          tunnel: [w640 w646] -> w633
          frame "Tunnel Speed", Default {
            n253 = local read "New Calib Filenames"() -> (w643:path[])
            n254 = Index Array(array=w643, index=0 ("Index")) -> (element=w644:path)
            n255 = call "Calibration.vi"("Mode"=Calib_mode."Take a New Calibration Point", "Calib file"=w644) -> ("Coefficients"=w640:dbl[][], "Status Out"=w642:T2)  [unwired: 1 in, 15 out]
          }
          frame "Concentration" {
            # "St Dev"
            # "Mean"
            n256 = stacked-sequence {
              seq-local: [_ w652 _] -> [_ _ w698]
              seq-local: [_ w651 _] -> [_ _ w697]
              tunnel: w648 -> [_ w655 _]
              tunnel: [_ w653 _] -> w647
              tunnel: [_ _ w699] -> w646
              frame #0 {
                n257 = global write "Meas_global.vi" "Remote control"(TRUE ("Remote control")) -> ()
                n258 = global write "Meas_global.vi" "Raw data option"(enum16{"Save raw data", "Raw data not saved"}."Save raw data" ("Raw data option")) -> ()
              }
              frame #1 {
                n259 = local read "New Calib Filenames"() -> (w656:path[])
                n260 = Index Array(array=w656, index=0 ("Index")) -> (element=w654:path)
                n261 = while {
                  tunnel: [w664] -> w653
                  tunnel: w654 -> [w663]
                  tunnel: w655 -> [w661]
                  tunnel: [w660] -> w652
                  tunnel: [w659] -> w651
                  i -> [w658]
                  stop <- w662 continue-if-true
                  n262 = stacked-sequence {
                    seq-local: [_ w667 _ _] -> [_ _ _ w691]
                    seq-local: [_ _ w676 _] -> [_ _ _ w695]
                    tunnel: [_ w667 _ _] -> w664
                    tunnel: w663 -> [_ w672 _ _]
                    tunnel: [_ _ _ w686] -> w662
                    tunnel: w661 -> [_ w668 _ _]
                    tunnel: [_ _ w677 _] -> w660
                    tunnel: [_ _ w676 _] -> w659
                    tunnel: w658 -> [_ _ _ w693]
                    frame #0 {
                      n263 = global write "Meas_global.vi" "Remote control"(TRUE ("Remote control")) -> ()
                    }
                    frame #1 {
                      n264 = call "Get_Data_Base_file_code.vi"("Data Type"="Raw_Calibrations", "Results Filename"=w672, "Short_Name"="Raw_Cal" ("Data Type")) -> ("Raw Data File Name"=w669:path)  [unwired: 1 in, 3 out]
                      n265 = call "Measurement.vi"("setup"=Setup."Run Program", "Post Process"=Post_Process."Take New Data", "File"=Save_Data."Save No Data", "Raw data file"=w669, "Setup filename"=w668) -> ("Status Out"=w667:T2)  [unwired: 2 in, 12 out]
                    }
                    frame #2 {
                      n266 = local read "FF Indexes"() -> (w678:i16[])
                      n267 = global read "Meas_global.vi" "Time Trace"() -> (w675:T23[])
                      n268 = for {
                        tunnel: w678 -> [w685] mode=indexing
                        tunnel: [w684] -> w677 mode=indexing
                        tunnel: [w683] -> w676 mode=indexing
                        tunnel: w675 -> [w681]
                        n269 = Index Array(array=w681, index=w685) -> (element=w680:T23)
                        n270 = Unbundle By Name(w680) -> ("Eng Values"=w679:dbl[])
                        n271 = call "De-spiked_Stats.vi"("Raw Signal"=w679, "No of st dev to chop at"=6.0) -> ("mean"=w684:dbl, "standard deviation"=w683:dbl)  [unwired: 1 out]
                      }
                    }
                    frame #3 {
                      n272 = Greater?(x=w695, y=0.15) -> (0:w694:bool[])
                      n273 = Or Array Elements(Boolean array=w694) -> (logical OR=w688:bool)
                      n274 = Less?(x=w693, y=2) -> (x < y?=w689:bool)
                      n275 = Equal?(x=w691, y=Multi_Run_Status."Continue" ("Status Out")) -> (x = y?=w687:bool)
                      n276 = Compound Arithmetic op=AND(w687, w688, w689) -> (w686:bool)
                    }
                  }
                }
              }
              frame #2 {
                n277 = local read "FFID St Dev"() -> (w702:dbl[][])
                n278 = local read "Valve position"() -> (w706:dbl)
                n279 = local read "Concentrations"() -> (w700:dbl[])
                n280 = global read "Meas_global.vi" "Temp"() -> (w707:dbl)
                n281 = Build Array (concatenate)(w698, w697) -> (w701:dbl[])
                n282 = Build Array (concatenate)(w702, w701) -> (→"FFID St Dev":dbl[][])
                n283 = Index Array(array=w700, index=w706) -> (element=w705:dbl)
                n284 = local read "New Calib Filenames"() -> (w704:path[])
                n285 = for {
                  tunnel: w698 -> [w713] mode=indexing
                  tunnel: w707 -> [w712]
                  tunnel: w705 -> [w711]
                  tunnel: [w710] -> w699 mode=indexing
                  tunnel: w704 -> [w709] mode=indexing
                  tunnel: w697 -> [w708] mode=indexing
                  n286 = stacked-sequence {
                    tunnel: w713 -> [w719 _]
                    tunnel: w712 -> [w716 _]
                    tunnel: w711 -> [w718 _]
                    tunnel: [_ w721] -> w710
                    tunnel: w709 -> [_ w720]
                    tunnel: w708 -> [w714 _]
                    frame #0 {
                      n287 = Build Array(w718, w719, w714, 0.0 ("element"), w716) -> (w717:dbl[])
                      n288 = global write "Calib_global.vi" "Calibration Points"(w717) -> ()
                    }
                    frame #1 {
                      n289 = call "Calibration.vi"("Mode"=Calib_mode."Refit Curve", "Calib file"=w720) -> ("Coefficients"=w722:dbl[][])  [unwired: 1 in, 16 out]
                      n290 = Index Array(array=w722, index (row)=0 ("Index")) -> (element=w721:dbl[])  [unwired: 1 in]
                    }
                  }
                }
              }
            }
          }
        }
        "Coefficients" <- w633
        n291 = local write "Status"(w634) -> ()
      }
      frame "Do Another Calibration Point?" {
        n292 = local read "No of Calib Points"() -> (w738:i32)
        n293 = local read "Status"() -> (w734:T2)
        n294 = local read "Currently On"() -> (w730:i32)
        n295 = case shown="\"Terminate Run\"" w734 {
          tunnel: [w748 w749 TRUE w752] -> w736
          tunnel: [w748 w749 FALSE w752] -> w737
          frame "Continue", Default {
            w748 = TRUE
          }
          frame "Jump to Next Point" {
            w749 = TRUE
          }
          frame "Jump to Next Row" {
          }
          frame "Terminate Run" {
            w752 = FALSE
          }
        }
        n296 = Greater?(x=w738, y=w730) -> (0:w735:bool)
        n297 = Compound Arithmetic op=AND(invert "stop", w736) -> (w733:bool)
        n298 = Compound Arithmetic op=AND(w733, w737, w735) -> (w731:bool)
        n299 = case shown="False" w731 {
          tunnel: w730 -> [_ w747]
          tunnel: [w741 Auto_Calib_Case."Set Measurement Conditions" ("Currently in Case")] -> w729
          tunnel: w728 -> [w742 _]
          tunnel: w727 -> [w740 _]
          frame False {
            n300 = case shown="\"Check VI only\"" w742 {
              tunnel: [Auto_Calib_Case."End" ("Currently in Case") Auto_Calib_Case."Skip Next Frame?" ("Currently in Case")] -> w741
              tunnel: w740 -> [_ _]
              frame "Check VI only" {
              }
              frame "Run VI" {
              }
            }
          }
          frame True {
            n301 = Increment(x=w747) -> (x+1=w746:i32)
            n302 = local write "Currently On"(w746) -> ()
          }
        }
        n303 = case shown="True" "stop" {
          frame False {
          }
          frame True {
            n304 = local write "Status"(Multi_Run_Status."Terminate Run" ("Status")) -> ()
          }
        }
      }
      frame "Skip Next Frame?" {
        n305 = local read "Status"() -> (w756:T2)
        n306 = case shown="\"Concentration\"" w753 {
          frame "Tunnel Speed", Default {
          }
          frame "Concentration" {
            w759 = T22 1 items=["", "Zero Air", "Calib 1", "Calib 2", "Measure"] ("Requested Position")
            n307 = call "Fast_FID_Valve_Control.vi"("Requested Position"=w759) -> ()  [unwired: 7 out]
          }
        }
        n308 = case shown="\"Continue\"" w756 {
          tunnel: [w760 Auto_Calib_Case."End" ("Currently in Case")] -> w755
          tunnel: w754 -> [w760 _]
          frame "Continue" {
          }
          frame "Terminate Run", Default {
          }
        }
      }
      frame "Insert New calibration Filenames into Measurement Setup file" {
        n309 = local read "New Calib Filenames"() -> (w762:path[])
        n310 = global read "Meas_global.vi" "Raw data file"() -> (w772:path)
        n311 = local read "Ch No's"() -> (w763:i16[])
        n312 = Strip Path(path=w772) -> (stripped path=w771:path)  [unwired: 1 out]
        n313 = Equal?(x=Auto_Calib_Type."Concentration" ("Calibration varying"), y=w769) -> (x = y?=w768:bool)
        n314 = call "Current_Calib_Filenames.vi"("Calib Filename"=w762, "Channel Numbers"=w763, "Mode"=App_Global."Write to Global") -> ()  [unwired: 3 out]
        n315 = case shown="False" w768 {
          tunnel: [Auto_Calib_Case."Warn if Current Calibration fit is poor" ("Currently in Case") w779] -> w767
          tunnel: w766 -> [_ w779]
          tunnel: w762 -> [_ w778]
          tunnel: [1 w777] -> w765
          frame False {
          }
          frame True {
            n316 = Array Size(array=w778) -> (size(s)=w777:i32)
          }
        }
        n317 = for {
          N: w765 -> [_]
          tunnel: w762 -> [w781] mode=indexing
          tunnel: w771 -> [w785]
          w783 = FALSE  # Variable Target?
          n318 = Strip Path(path=w781) -> (name=w784:string)  [unwired: 1 out]
          n319 = Build Path(base path=w785, name or relative path=w784) -> (appended path=w780:path)
          n320 = call "Remember_Calib_Filenames.vi"("Filename to Remember"=w780) -> ()  [unwired: 1 out]
          n321 = call "Copy_with_Check.vi"("Mode"=enum16{"Move", "Copy"}."Copy", "Target Path"=w780, "Variable Target?"=w783, "Source Path"=w781) -> ()  [unwired: 1 out]
        }
      }
      frame "Warn if FFID calibration is very non linear" {
        w802 = FALSE  # Dialog Box (T)
        n322 = local read "Root Name"() -> (w801:string[])
        n323 = local read "Coefficients"() -> (w804:dbl[][])
        n324 = for {
          tunnel: w804 -> [w811] mode=indexing
          shift-right: [w813] -> w799
          shift-left: "" -> [w814]
          tunnel: w801 -> [w815] mode=indexing
          tunnel: [w808] -> w794 mode=indexing
          tunnel: "If the calibration fit for %s had been linear instead of a second order polynomial, it would have yielded an average fit error of %.1f%%.\\n" ("Format String") -> [w806]
          n325 = Index Array(array=w811, index=0 ("Index")) -> (element=w809:dbl)
          n326 = Absolute Value(x=w809) -> (abs(x)=w808:dbl)
          n327 = Less?(x=w808, y=2.2) -> (x < y?=w812:bool)
          n328 = case shown="False" w812 {
            tunnel: w815 -> [w817 _]
            tunnel: w808 -> [w818 _]
            tunnel: w814 -> [w821 w822]
            tunnel: [w819 w822] -> w813
            tunnel: w806 -> [w816 _]
            frame False {
              n329 = Format Into String(format string=w816, w817, w818) -> (resulting string=w820:string)  [unwired: 2 in, 1 out]
              n330 = Concatenate Strings(w821, w820) -> (w819:string)
            }
            frame True {
            }
          }
        }
        n331 = Array Max & Min(array=w794) -> (max value=w793:dbl)  [unwired: 3 out]
        n332 = Greater?(x=w793, y=7.0) -> (0:w791:bool)
        n333 = Select(t="Very Poor FFID Linearity", s=w791, f="Poor FFID Linearity") -> (s? t:f=w788:string)
        n334 = Empty String/Path?(string/path=w799) -> (empty?=w798:bool)
        n335 = Not(x=w798) -> (.not. x?=w797:bool)
        n336 = Bundle By Name(cluster=errorcluster {"status"=FALSE, "code"=0, "source"=""} ("error in (no error)"), "source"=w799, "status"=w797) -> (w796:errorcluster)
        n337 = call "EnFlo_Error_Handler.vi"("error in (no error)"=w796, "Error Type"=w788, "Dialog Box (T)"=w802) -> ()  [unwired: 3 out]
      }
      frame "Warn if FFID variance is high" {
        w844 = FALSE  # Dialog Box (T)
        n338 = local read "New Calib Filenames"() -> (w826:path[])
        n339 = local read "FFID St Dev"() -> (w846:dbl[][])
        n340 = Index Array(array=w831, index (col)=0 ("disabled index (col)")) -> (element=w829:dbl[])  [unwired: 1 in]
        n341 = Array Size(array=w826) -> (size(s)=w825:i32)
        n342 = for {
          tunnel: w846 -> [w863]
          shift-right: [w865] -> w842
          shift-left: "" -> [w866]
          tunnel: w826 -> [w854] mode=indexing
          tunnel: "For %s the measurement at %dppm had a standard deviation of %.2f volts for an average value of  %.1f volts.\\n" ("Format String") -> [w864]
          tunnel: w829 -> [w857]
          tunnel: [w856] -> w827 mode=indexing
          tunnel: w825 -> [w852]
          tunnel: [w848] -> w823 mode=indexing
          i -> [w851]
          n343 = Add(x=w852, y=w851) -> (x+y=w850:i32)
          n344 = Strip Path(path=w854) -> (name=w853:string)  [unwired: 1 out]
          n345 = Index Array(array=w863, index (col)=w851) -> (element=w855:dbl[])  [unwired: 1 in]
          n346 = Index Array(array=w863, index (col)=w850) -> (element=w849:dbl[])  [unwired: 1 in]
          n347 = Array Max & Min(array=w849) -> (min value=w848:dbl)  [unwired: 3 out]
          n348 = call-poly <vilib>:"Mean.vi"("X"=w855) -> ("mean"=w862:dbl)  [unwired: 1 out]
          n349 = Divide(x=w849, y=w862) -> (x/y=w861:dbl[])
          n350 = Array Max & Min(array=w861) -> (max value=w856:dbl, max index (indices)=w858:i32)  [unwired: 2 out]
          n351 = Greater?(x=w856, y=0.06) -> (0:w859:bool)
          n352 = case shown="True" w859 {
            tunnel: w853 -> [_ w877]
            tunnel: w866 -> [w867 w883]
            tunnel: [w867 w881] -> w865
            tunnel: w864 -> [_ w880]
            tunnel: w858 -> [_ w878]
            tunnel: w857 -> [_ w879]
            tunnel: w856 -> [_ _]
            tunnel: w849 -> [_ w876]
            tunnel: w855 -> [_ w874]
            frame False {
            }
            frame True {
              n353 = local read "Concentrations"() -> (w872:dbl[])
              n354 = Index Array(array=w879, index=w878) -> (element=w873:dbl)
              n355 = Index Array(array=w876, index=w878) -> (element=w870:dbl)
              n356 = Index Array(array=w874, index=w878) -> (element=w875:dbl)
              n357 = Index Array(array=w872, index=w873) -> (element=w871:dbl)
              n358 = Multiply(x=w870, y=2.5) -> (x*y=w869:dbl)
              n359 = Format Into String(format string=w880, w877, w871, w869, w875) -> (resulting string=w882:string)  [unwired: 2 in, 1 out]
              n360 = Concatenate Strings(w883, w882) -> (w881:string)
            }
          }
        }
        "Minimum St Dev" <- w823
        n361 = Array Max & Min(array=w827) -> (max value=w837:dbl)  [unwired: 3 out]
        n362 = Greater?(x=w837, y=0.09) -> (0:w835:bool)
        n363 = Select(t="Very unstable FFID calibration point", s=w835, f="Unstable FFID calibration point") -> (s? t:f=w832:string)
        n364 = Empty String/Path?(string/path=w842) -> (empty?=w841:bool)
        n365 = Not(x=w841) -> (.not. x?=w840:bool)
        n366 = Bundle By Name(cluster=errorcluster {"status"=FALSE, "code"=0, "source"=""} ("error in (no error)"), "source"=w842, "status"=w840) -> (w839:errorcluster)
        n367 = call "EnFlo_Error_Handler.vi"("error in (no error)"=w839, "Error Type"=w832, "Dialog Box (T)"=w844) -> ()  [unwired: 3 out]
      }
      frame "Insert Bkgnd Variance into calib file" {
        n368 = local read "New Calib Filenames"() -> (w886:path[])
        n369 = local read "Minimum St Dev"() -> (w887:dbl[])
        n370 = local read "Coefficients"() -> (w884:dbl[][])
        n371 = for {
          tunnel: w887 -> [w892] mode=indexing
          tunnel: w886 -> [w898] mode=indexing
          tunnel: w884 -> [w895] mode=indexing
          n372 = call "Read_File_Simple.vi"("Filename"=w898) -> ("string"=w902:string)  [unwired: 2 in, 7 out]
          n373 = Index Array(array=w895, index=2) -> (element=w893:dbl)
          n374 = Multiply(x=w892, y=w893) -> (x*y=w891:dbl)
          n375 = Square(x=w891) -> (x^2=w890:dbl)
          n376 = Number To Fractional String(number=w890, precision (6)=i16 8) -> (F-format string=w900:string)  [unwired: 2 out]
          n377 = call "Replace_data_in_setup_string.vi"("New data string"=w900, "Input string"=w902, "Variable name"="Fast FID Bkgnd Variance") -> ("Appended string"=w897:string)
          n378 = call "Write_File_Simple.vi"("append to file? (new file:F)"=FALSE, "character string"=w897, "file path"=w898) -> ()  [unwired: 2 out]
        }
      }
      frame "Warn if FFID voltages are too low" {
        w920 = FALSE  # Dialog Box (T)
        n379 = local read "Coefficients"() -> (w910:dbl[][])
        n380 = local read "Concentrations"() -> (w906:dbl[])
        n381 = Index Array(array=w913, index (col)=0 ("disabled index (col)")) -> (element=w905:dbl[])  [unwired: 1 in]
        n382 = local read "New Calib Filenames"() -> (w909:path[])
        n383 = for {
          tunnel: w906 -> [w925]
          tunnel: w905 -> [w924] mode=indexing
          tunnel: [w923] -> w904 mode=indexing
          n384 = Index Array(array=w925, index=w924) -> (element=w923:dbl)
        }
        n385 = Array Max & Min(array=w904) -> (max value=w903:dbl)  [unwired: 3 out]
        n386 = for {
          shift-right: [w935] -> w918
          shift-left: "" -> [w936]
          tunnel: "For %s the maximum measured calibration voltage was %.1f volts.\nCheck that the FID is running and correctly connected to the acquisition system." ("Format String") -> [w934]
          tunnel: w910 -> [w932] mode=indexing
          tunnel: w909 -> [w928] mode=indexing
          tunnel: w903 -> [w927]
          n387 = Split 1D Array(array=w932, index=1) -> (second subarray=w931:dbl[])  [unwired: 1 out]
          n388 = call "Polybackwards.vi"("Coefficients"=w931, "Y input"=w927) -> ("X output"=w926:dbl)  [unwired: 1 out]
          n389 = Less?(x=w926, y=0.2) -> (x < y?=w929:bool)
          n390 = case shown="True" w929 {
            tunnel: w936 -> [w937 w944]
            tunnel: [w937 w942] -> w935
            tunnel: w934 -> [_ w941]
            tunnel: w928 -> [_ w940]
            tunnel: w926 -> [_ w938]
            frame False {
            }
            frame True {
              n391 = Strip Path(path=w940) -> (name=w939:string)  [unwired: 1 out]
              n392 = Format Into String(format string=w941, w939, w938) -> (resulting string=w943:string)  [unwired: 2 in, 1 out]
              n393 = Concatenate Strings(w944, w943) -> (w942:string)
            }
          }
        }
        n394 = Empty String/Path?(string/path=w918) -> (empty?=w917:bool)
        n395 = Not(x=w917) -> (.not. x?=w916:bool)
        n396 = Bundle By Name(cluster=errorcluster {"status"=FALSE, "code"=0, "source"=""} ("error in (no error)"), "source"=w918, "status"=w916) -> (w915:errorcluster)
        n397 = call "EnFlo_Error_Handler.vi"("error in (no error)"=w915, "Error Type"="Low FFID calibration voltages", "Dialog Box (T)"=w920) -> ()  [unwired: 3 out]
      }
      frame "Warn if Current Calibration fit is poor" {
        w959 = FALSE  # Dialog Box (T)
        n398 = local read "Root Name"() -> (w958:string[])
        n399 = local read "Coefficients"() -> (w961:dbl[][])
        n400 = for {
          tunnel: w961 -> [w968] mode=indexing
          shift-right: [w970] -> w956
          shift-left: "" -> [w971]
          tunnel: w958 -> [w972] mode=indexing
          tunnel: [w965] -> w951 mode=indexing
          n401 = Index Array(array=w968, index=0 ("Index")) -> (element=w966:dbl)
          n402 = Absolute Value(x=w966) -> (abs(x)=w965:dbl)
          n403 = Less?(x=w965, y=1.0) -> (x < y?=w969:bool)
          n404 = case shown="True" w969 {
            tunnel: w972 -> [w974 _]
            tunnel: w965 -> [w975 _]
            tunnel: w971 -> [w978 w979]
            tunnel: [w976 w979] -> w970
            frame False {
              n405 = Format Into String(format string="The calibration for %s has an average fit error of %.1f%%\\n" ("Format String"), w974, w975) -> (resulting string=w977:string)  [unwired: 2 in, 1 out]
              n406 = Concatenate Strings(w978, w977) -> (w976:string)
            }
            frame True {
            }
          }
        }
        n407 = Array Max & Min(array=w951) -> (max value=w950:dbl)  [unwired: 3 out]
        n408 = Greater?(x=w950, y=7.0) -> (0:w948:bool)
        n409 = Select(t="Very Poor Calibration", s=w948, f="Poor Calibration") -> (s? t:f=w945:string)
        n410 = Empty String/Path?(string/path=w956) -> (empty?=w955:bool)
        n411 = Not(x=w955) -> (.not. x?=w954:bool)
        n412 = Bundle By Name(cluster=errorcluster {"status"=FALSE, "code"=0, "source"=""} ("error in (no error)"), "source"=w956, "status"=w954) -> (w953:errorcluster)
        n413 = call "EnFlo_Error_Handler.vi"("error in (no error)"=w953, "Error Type"=w945, "Dialog Box (T)"=w959) -> ()  [unwired: 3 out]
      }
      frame "Warn if Calibration Coefficients have significantly altered" {
        w1005 = FALSE  # Dialog Box (T)
        w992 = 8.0 ("y")
        n414 = local read "New Calib Filenames"() -> (w997:path[])
        n415 = local read "Root Name"() -> (w996:string[])
        n416 = global read "Calib_global.vi" "Instrument type"() -> (w995:T14)
        n417 = Unbundle By Name(w984) -> ("Extra Commands"=w983:string)
        n418 = global read "Extra_Commands_Global.vi" "If Command"() -> (w985:string)
        n419 = call "Extra_Commands.vi"("String to Search"=w983, "Command"=w985) -> ("String Value"=w982:string)  [unwired: 1 in, 4 out]
        n420 = call "Calibration_Analysis.vi"("Root Name"=w996, "New Calib Filenames"=w997, "Instrument type"=w995, "Clear Calib History"="Clear Calib History") -> ("Error String"=w994:string, "Max % Error"=w980:dbl)
        n421 = call "Get_array_values_fr_String.vi"("String Value"=w982) -> ("Numeric Array"=w981:dbl[], "String array"=w987:string[])
        n422 = Greater?(x=w980, y=w992) -> (0:w993:bool)
        n423 = Index Array(array=w987, index=0 ("Index")) -> (element=w988:string)
        n424 = case shown="\"Drift Greater Than\"" w988 {
          tunnel: w981 -> [w1011 _]
          tunnel: w980 -> [w1010 _]
          frame "Drift Greater Than" {
            n425 = Index Array(array=w1011, index=1 ("Index")) -> (element=w1009:dbl)
            n426 = Greater?(x=w1010, y=w1009) -> (0:w1008:bool)
            n427 = case shown="True" w1008 {
              frame False {
              }
              frame True {
                n428 = local write "Status"(Multi_Run_Status."Jump To Fall Back" ("Status")) -> ()
              }
            }
          }
          frame "No Match", Default {
          }
        }
        n429 = Format Into String(format string="Calibration Drift Greater than %d%%", w992) -> (resulting string=w990:string)  [unwired: 2 in, 1 out]
        n430 = Select(t=w990, s=w993, f="Calibration Drift") -> (s? t:f=w998:string)
        n431 = Empty String/Path?(string/path=w994) -> (empty?=w1003:bool)
        n432 = Not(x=w1003) -> (.not. x?=w1002:bool)
        n433 = Bundle By Name(cluster=errorcluster {"status"=FALSE, "code"=0, "source"=""} ("error in (no error)"), "source"=w994, "status"=w1002) -> (w1001:errorcluster)
        n434 = call "EnFlo_Error_Handler.vi"("error in (no error)"=w1001, "Error Type"=w998, "Dialog Box (T)"=w1005) -> ()  [unwired: 3 out]
      }
      frame "End" {
        n435 = case shown="\"Concentration\"" w1017 {
          tunnel: w1015 -> [_ w1023]
          tunnel: w1016 -> [_ w1021]
          tunnel: w1014 -> [_ w1022]
          frame "Tunnel Speed", Default {
          }
          frame "Concentration" {
            n436 = stacked-sequence {
              tunnel: w1023 -> [w1040 _]
              tunnel: w1022 -> [w1039 _]
              tunnel: w1021 -> [w1028 w1047]
              frame #0 {
                n437 = Unbundle By Name(w1040) -> ("Averaging time (min)"=w1042:dbl)
                n438 = global read "Trav_pos_global.vi" "Simulation Time"() -> (w1031:timestamp)
                n439 = Unbundle By Name(w1040) -> ("Start X"=w1026:dbl, "Start Z"=w1027:dbl)
                n440 = Select(t=3 ("No. of pts."), s=w1039, f=2 ("No. of pts.")) -> (s? t:f=w1033:i32)
                n441 = Multiply(x=60.0, y=w1042) -> (x*y=w1036:dbl)
                n442 = Add(x=w1026, y=6.0) -> (x+y=w1025:dbl)
                n443 = Add(x=w1027, y=150.0) -> (x+y=w1043:dbl)
                n444 = Add(x=w1036, y=60.0) -> (x+y=w1034:dbl)
                n445 = Bundle By Name(cluster=w1040, "Start X"=w1025, "Start Z"=w1043) -> (w1044:T5)
                n446 = Multiply(x=w1034, y=w1033) -> (x*y=w1032:dbl)
                n447 = Add(x=w1031, y=w1032) -> (x+y=w1029:timestamp)
                n448 = call "Set_Traverse_Position.vi"("Simulate/Run"=w1028, "Currently on Point"=1, "Traverse line"=w1044) -> ()  [unwired: 3 out]
                n449 = call "Run_FFID_Bkgnd.vi"("Simulated Time"=w1029, "Run Now?"=TRUE, "Simulate/Run"=w1028) -> ()  [unwired: 3 out]
              }
              frame #1 {
                n450 = case shown="\"Run VI\"" w1047 {
                  frame "Check VI only", Default {
                  }
                  frame "Run VI" {
                    w1048 = T22 4 items=["", "Zero Air", "Calib 1", "Calib 2", "Measure"] ("Requested Position")
                    n451 = call "Fast_FID_Valve_Control.vi"("Requested Position"=w1048) -> ()  [unwired: 7 out]
                  }
                }
              }
            }
          }
        }
      }
    }
    "Currently in Case" <- w17
  }
  "Error Messages" <- w11
